vi "NiFPGA Read FIFO - I16.vi"(6 "Timeout":u32, 8 "error in (no error)":errorcluster, 9 "Number of Elements":u32, 10 "FIFO":u32, 11 "Session":u32) -> (0 "error out":errorcluster, 1 "Data":i16[](array[numeric]), 3 "Session Out":u32, 4 "Elements Remaining":u32)   [LabVIEW 2010, in "FPGA Interface Wrapper.lvlib"]
doc: "Reads from a FIFO of signed 16-bit integers."
uses:
  <userlib>/_FPGA Interface Advanced Tools/FPGA Interface Wrapper/FPGA Interface Wrapper.lvlib
  NiFpga.dll
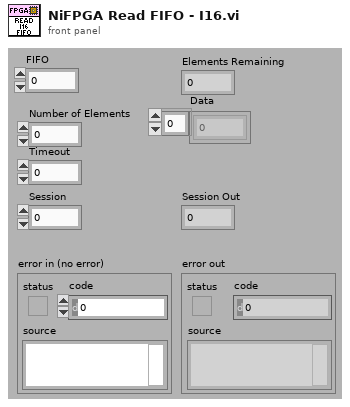
[diagram p1: front panel]
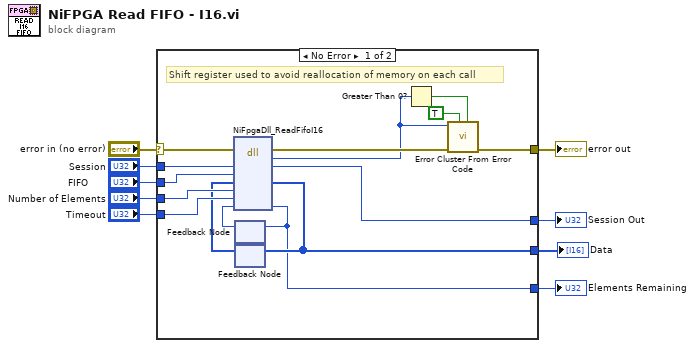
[diagram p0: block diagram]
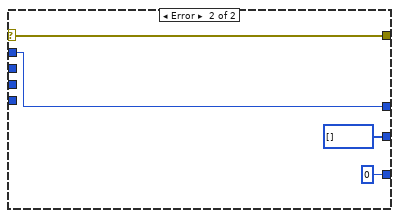
[diagram p2: hidden frame]
diagram:
  n1 = case shown="No Error" "error in (no error)" {
    selector: "error in (no error)" -> [w24 w27]
    tunnel: [w15 w27] -> w8
    tunnel: "Session" -> [w23 w28]
    tunnel: [w22 w28] -> w6
    tunnel: "FIFO" -> [w21 _]
    tunnel: "Number of Elements" -> [w20 _]
    tunnel: "Timeout" -> [w19 _]
    tunnel: [w10 u64 0 ("Elements Remaining")] -> w2
    tunnel: [w11 i16[] [] ("Data")] -> w1
    frame No Error {
      # "Shift register used to avoid reallocation of memory on each call"
      n2 = feedback #1() -> (w12:u64)  [unwired: 1 in]
      n3 = feedback #2() -> (w13:i16[])  [unwired: 1 in]
      n4 = dll-call lib="NiFpga.dll" fn="NiFpgaDll_ReadFifoI16"(error in=w24, "Session"=w23, "FIFO"=w21, "Data"=w13, "Number of Elements"=w20, "Timeout"=w19, "Elements Remaining"=w12) -> (error out=w16:errorcluster, "Status"=w14:i32, "Session"=w22:u32, "Data"=w11:i16[], "Elements Remaining"=w10:u64)  [unwired: 5 in, 1 out]
      n5 = feedback-in #1(w10) -> ()
      n6 = feedback-in #2(w11) -> ()
      n7 = Greater Than 0?(x=w14) -> (x > 0?=w17:bool)
      n8 = call <vilib>:"Error Cluster From Error Code.vi"("is warning? (False)"=w17, "show call chain? (False)"=TRUE, "error in (no error)"=w16, "error code (0)"=w14) -> ("error out"=w15:errorcluster)  [unwired: 5 in]
    }
    frame Error {
    }
  }
  "error out" <- w8
  "Session Out" <- w6
  "Elements Remaining" <- w2
  "Data" <- w1
